vi "ResizeObjectsInAllPanes.vi"(8 "error in (no error)":errorcluster, 11 "PentaPanesGUI in":refnum<class "PentaPanes.lvclass">) -> (0 "error out":errorcluster, 3 "PentaPanesGUI out":refnum<class "PentaPanes.lvclass">)   [LabVIEW 2022 SP3, in "PentaPanesLibrary.lvlib" / "PentaPanes.lvclass"]
uses:
  PentaPanes.lvclass
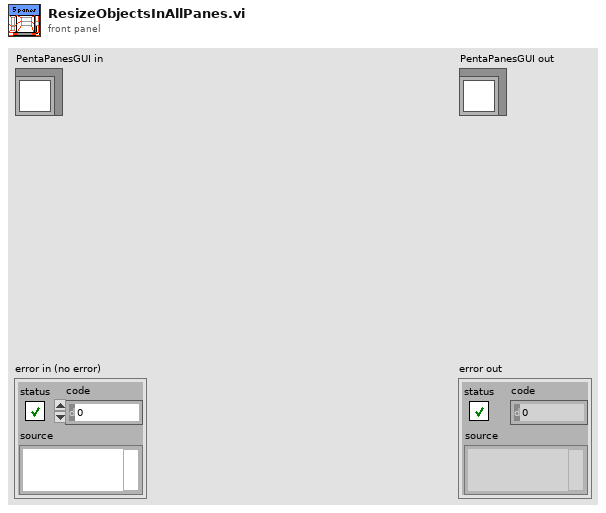
[diagram p1: front panel]
types:
  T1 = typedef "PentaPanesLibrary.lvlib/PentaPanes.lvclass/PanesCluster.ctl" = cluster{"Top Pane":refnum<vi>, "Left Pane":refnum<vi>, "Center Pane":refnum<vi>, "Right Pane":refnum<vi>, "Bottom Pane":refnum<vi>}
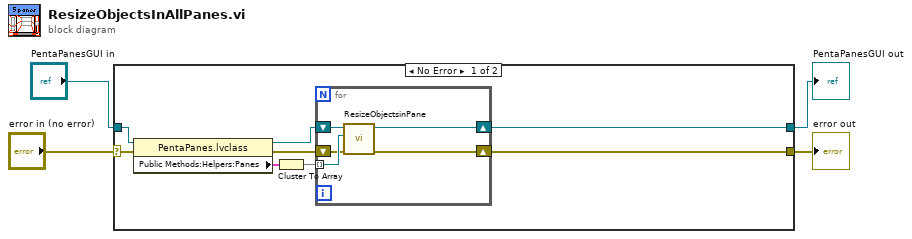
[diagram p0: block diagram]
diagram:
  n1 = case shown="No Error" "error in (no error)" {
    selector: "error in (no error)" -> [w6 w19]
    tunnel: [w5 w19] -> w3
    tunnel: [w7 w18] -> w1
    tunnel: "PentaPanesGUI in" -> [w8 w18]
    frame No Error {
      n2 = property class="PentaPanes.lvclass"(reference=w8, error in=w6) -> (reference out=w11:refnum<class "PentaPanes.lvclass">, error out=w12:errorcluster, "Public Methods:Helpers:Panes"=w9:T1)
      n3 = Cluster To Array(cluster=w9) -> (array=w10:refnum<vi>[])
      n4 = for {
        tunnel: w10 -> [w17] mode=indexing
        shift-right: [w15] -> w7
        shift-left: w11 -> [w16]
        shift-right: [w13] -> w5
        shift-left: w12 -> [w14]
        n5 = call-dynamic "ResizeObjectsinPane.vi"("error in (no error)"=w14, "PaneRef"=w17, "PentaPanesGUI in"=w16) -> ("error out"=w13:errorcluster, "PentaPanesGUI out"=w15:refnum<class "PentaPanes.lvclass">)  [unwired: 7 in]
      }
    }
    frame Error {
    }
  }
  "error out" <- w3
  "PentaPanesGUI out" <- w1
